vi "amplitud_lookup.vi"(10 "theta_min":dbl, 11 "theta_max":dbl) -> (2 "amp1":dbl, 3 "amp3":dbl)   [LabVIEW 2013]
uses:
  <vilib>/Simulation/Implementation/Shared/SIMSCR Execution Mode.ctl
  <vilib>/Simulation/Scripting/Companion Diagram/SimConfigNode/SimParams.ctl
  <vilib>/Simulation/Scripting/Companion Diagram/SimConfigNode/_simSolvers.ctl
  <vilib>/Simulation/Param Hierarchy/Typedefs/SIMPH Param Control Actions.ctl
  <vilib>/Simulation/Implementation/Shared/NILVSim_ParamChanged.vi
  <vilib>/Simulation/Implementation/Shared/NILVSIM_BeginStep.vi
  <vilib>/Simulation/LookUpTables/Implementation/NILVSim LUT 1D.llb/SIM LUT 1D (scalar).vi
  <vilib>/Simulation/Implementation/Shared/NILVSim_Manager.vi
  <vilib>/Simulation/Implementation/Shared/NILVSim_FinalizeModel.vi
  <vilib>/Simulation/Implementation/Shared/SIM Unbundle Sim Info.vi
  <vilib>/Utility/error.llb/Clear Errors.vi
  <vilib>/Simulation/Implementation/Shared/NILVSim_GetModelError.vi
  <vilib>/Simulation/Implementation/Shared/SIM SimErrorHandler.vi
  <vilib>/Simulation/Implementation/Shared/SIM Bundle Sim Info.vi
  <vilib>/Simulation/Implementation/Shared/SIMSH Read Queue.vi
  <vilib>/Simulation/Implementation/Shared/NILVSim_Initialize.vi
  <vilib>/Simulation/Utility/Implementation/NILVSim Get Time and IsAcceptedStep.vi
  <vilib>/Simulation/Scripting/Companion Diagram/SimConfigNode/SimDog.xnode
  <vilib>/Simulation/Implementation/XNodeFramework/SimXNode/SimX.xnode
  <vilib>/Simulation/Implementation/Shared/NI_SIM_Implementation.lvlib
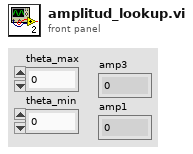
[diagram p1: front panel]
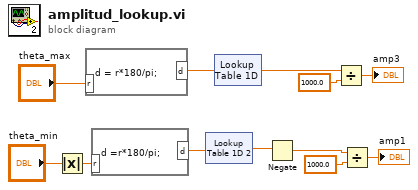
[diagram p0: block diagram]
diagram:
  n1 = Absolute Value(x="theta_min") -> (abs(x)=w4:dbl)
  n2 = formula code="d = r*180/pi;" ("Formula Node 2")("r"="theta_max") -> ("d"=w12:dbl)
  n3 = formula code="d =r*180/pi;"("r"=w4) -> ("d"=w1:dbl)
  n4 = xnode "Lookup Table 1D 2"("X Val"=w1) -> ("Result"=w2:dbl)  [unwired: 5 in]
  n5 = xnode "Lookup Table 1D"("X Val"=w12) -> ("Result"=w6:dbl)  [unwired: 5 in]
  n6 = Negate(x=w2) -> (-x=w5:dbl)
  n7 = Divide ("Divide 2")(x=w6, y=1000.0 ("y 2")) -> (x/y=→"amp3":dbl)
  n8 = Divide(x=w5, y=1000.0) -> (x/y=→"amp1":dbl)
